vi "cRIO Output voltage.vi"(5 "Voltage":dbl, 7 "AO Channel":string(combo)="AO0", 8 "error in (no error)":errorcluster, 11 "DAQ_CMD_Writer endpoint":refnum<k21>) -> (0 "error out":errorcluster, 3 "DAQ_CMD_Writer endpoint out":refnum<k21>)   [LabVIEW 2024]
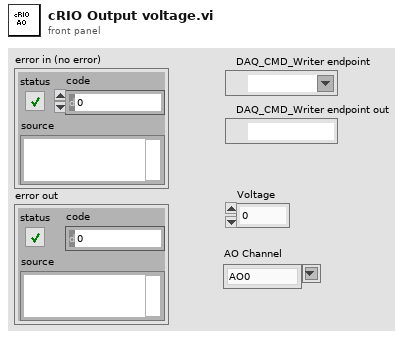
[diagram p1: front panel]
types:
  T1 = cluster{"Command":string, "Voltage":dbl, "Channel":string}
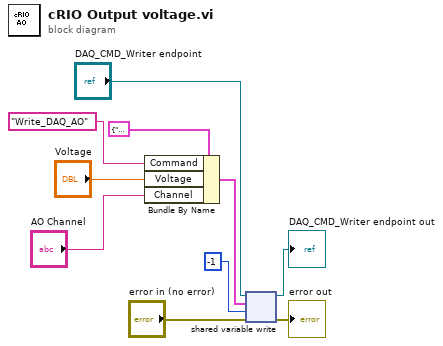
[diagram p0: block diagram]
diagram:
  n1 = Bundle By Name(cluster=T1 {"Command"="", "Voltage"=0.0, "Channel"=""} ("output cluster"), "Command"="Write_DAQ_AO", "Voltage"="Voltage", "Channel"="AO Channel") -> (w1:T1)
  n2 = shared-variable-write("DAQ_CMD_Writer endpoint", "error in (no error)", w1, -1 ("timeout ms (-1)")) -> (→"DAQ_CMD_Writer endpoint out":refnum<k21>, →"error out":errorcluster)  [unwired: 1 out]
